vi "Main.vi"() -> ()   [LabVIEW 2015]
doc: "Use this template to build a producer/consumer design pattern with events to produce queue items. Use this design pattern instead of the User Interface Event Handler pattern for user interfaces when you want to execute code asynchronously in response to an event without slowing the user interface responsiveness."
uses:
  Typedef/JSONCluster.ctl
  Typedef/Zone Data.ctl
  <vilib>/Rock Robotics/WPI/Camera/WPI_CameraSettings Read MJPG.ctl
  <vilib>/Rock Robotics/WPI/Camera/WPI_CameraImageSize.ctl
  <vilib>/LVH/i3 JSON/i3-json.lvlib
panel:
  in  "Match List":i32(listbox)
  out "Tab":enum32{"JSON", "Field", "Match"}(tab)
  in  "Autosave CSV":bool=TRUE
  out "JSON":string
  in  "JSON Tree":string(tree)
  in  "Field Setup":bool
  in  "Save As Button":bool
  in  "Save Button":bool
  in  "Scan":bool
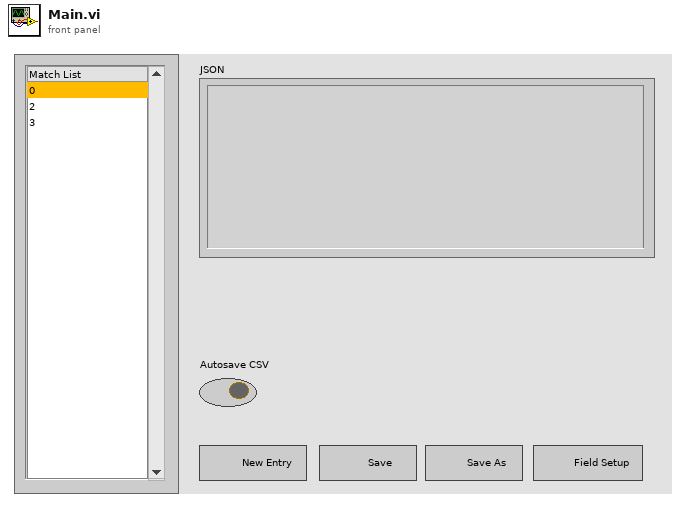
[diagram p1: front panel]
types:
  T1 = typedef "JSONCluster.ctl" = cluster{"preMatchData":cluster{"teamNumber":i32, "matchNumber":i32, "defenses":cluster{"blue1":string, "blue2":string, "blue3":string, "blue4":string, "blue5":string, "red1":string, "red2":string, "red3":string, "red4":string, "red5":string}}, "matchData":cluster{"name":string, "value":string, "items":cluster{"x":i32, "y":i32}[]}[], "matchComments":cluster{"matchComments":string, "lastComments":string}}
  T2 = typedef "Zone Data.ctl" = cluster{"Rect":cluster{"left":i16, "top":i16, "right":i16, "bottom":i16}, "Replace Values":cluster{"key":string, "value":string}[], "Name":string}
  T3 = cluster{"JSON":string, "JSONCluster":T1, "Cancelled":bool, "JSON Path":path, "CSV Path":path, "Zones":T2[]}
  T4 = typedef "WPI_CameraSettings Read MJPG.ctl" = cluster{"fps":i32, "compression":i32, "Image Size":T5}
  T5 = typedef "WPI_CameraImageSize.ctl" = enum16{"640x480", "320x240", "160x120", "Custom"}
  T6 = cluster{"teamNumber":i32, "matchNumber":i32, "defenses":cluster{"blue1":string, "blue2":string, "blue3":string, "blue4":string, "blue5":string, "red1":string, "red2":string, "red3":string, "red4":string, "red5":string}}
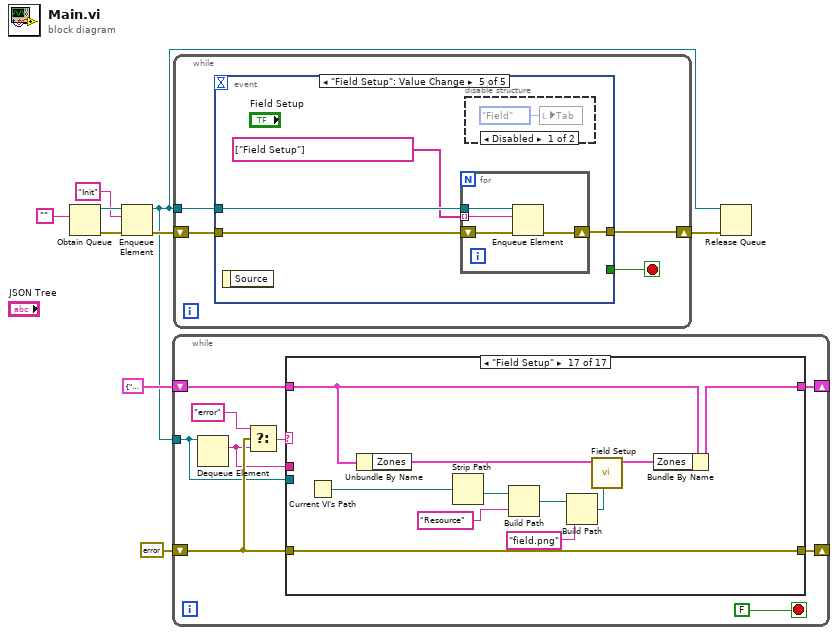
[diagram p0: block diagram]
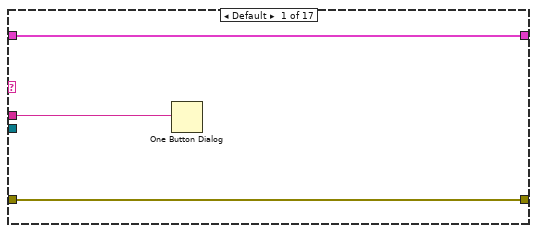
[diagram p2: hidden frame]
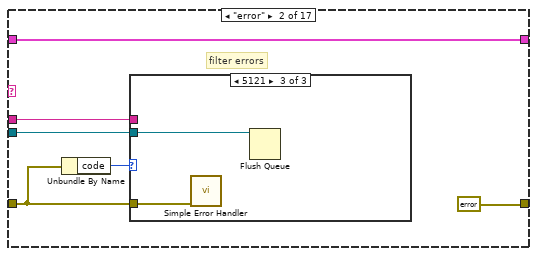
[diagram p3: hidden frame]
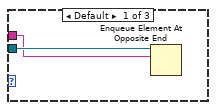
[diagram p4: hidden frame]
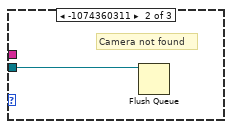
[diagram p5: hidden frame]
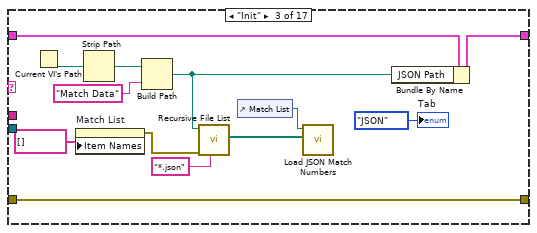
[diagram p6: hidden frame]
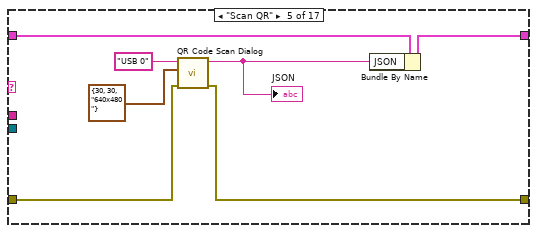
[diagram p8: hidden frame]
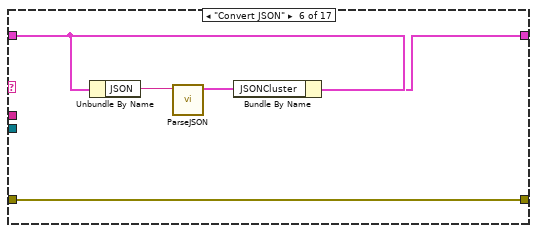
[diagram p9: hidden frame]
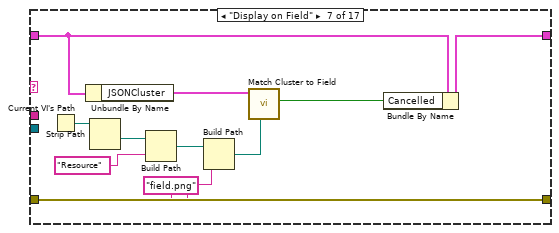
[diagram p10: hidden frame]
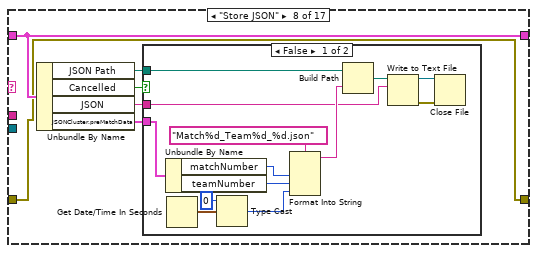
[diagram p11: hidden frame]
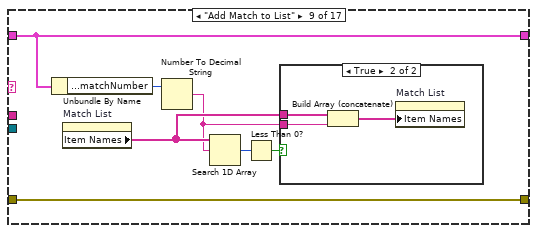
[diagram p13: hidden frame]
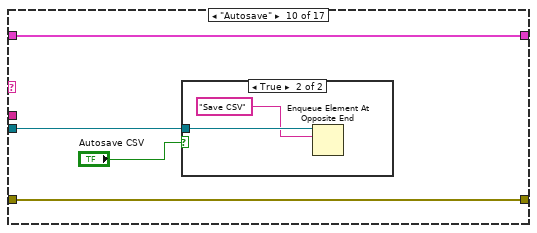
[diagram p15: hidden frame]
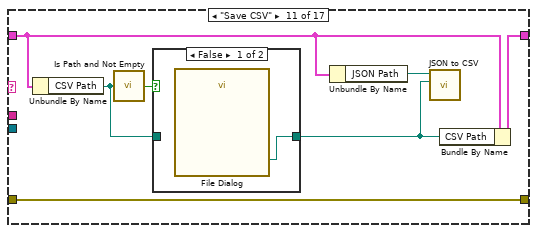
[diagram p17: hidden frame]
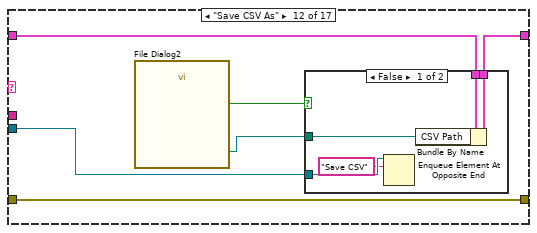
[diagram p19: hidden frame]
diagram:
  n1 = Obtain Queue(element data type="" ("data")) -> (queue out=w4:refnum<queue>, error out=w9:errorcluster)  [unwired: 4 in, 1 out]
  n2 = Enqueue Element(queue=w4, element="Init", error in (no error)=w9) -> (queue out=w3:refnum<queue>, error out=w5:errorcluster)  [unwired: 1 in, 1 out]
  n3 = while {
    tunnel: w3 -> [w10]
    shift-right: [w16] -> _
    shift-left: T3 {"JSON"="", "JSONCluster"={"preMatchData"={"teamNumber"=0, "matchNumber"=0, "defenses"={"blue1"="", "blue2"="", "blue3"="", "blue4"="", "blue5"="", "red1"="", "red2"="", "red3"="", "red4"="", "red5"=""}}, "matchData"=[], "matchComments"={"matchComments"="", "lastComments"=""}}, "Cancelled"=FALSE, "JSON Path"=path "", "CSV Path"=path "", "Zones"=[]} -> [w17]
    shift-right: [w13] -> _
    shift-left: errorcluster {"status"=FALSE, "code"=0, "source"=""} ("error out") -> [w12]
    stop <- FALSE stop-if-true
    n4 = Dequeue Element(queue=w10) -> (element=w11:string)  [unwired: 2 in, 3 out]
    n5 = Select(t="error", s=w12, f=w11) -> (s? t:f=w15:string)
    n6 = case shown="\"Field Setup\"" w15 {
      tunnel: w17 -> [w21 w27 w45 w47 w52 w58 w69 w76 w96 w103 w108 w119 w128 w138 w145 w147 w157]
      tunnel: [w21 w27 w44 w47 w51 w57 w68 w76 w96 w103 w107 w118 w128 w140 w145 w147 w155] -> w16
      tunnel: [w20 errorcluster {"status"=FALSE, "code"=0, "source"=""} ("error out") w38 w46 w49 w55 w66 w71 w90 w102 w112 w120 w127 w129 w142 w146 w158] -> w13
      tunnel: w12 -> [w20 w25 w38 w46 w48 w55 w66 w71 w90 w102 w112 w120 w127 w130 w143 w146 w158]
      tunnel: w11 -> [w19 w22 _ _ _ _ _ _ _ _ _ _ _ _ _ _ _]
      tunnel: w10 -> [_ w23 _ _ _ _ _ _ _ w101 _ w115 _ _ _ _ _]
      frame Default {
        n7 = One Button Dialog(message=w19) -> ()  [unwired: 1 in, 1 out]
      }
      frame "error" {
        # "filter errors"
        n8 = Unbundle By Name(w25) -> ("code"=w24:i32)
        n9 = case shown="5121" w24 {
          tunnel: w25 -> [_ _ w31]
          tunnel: w23 -> [w29 w30 w32]
          tunnel: w22 -> [w28 _ _]
          frame Default {
            n10 = Enqueue Element At Opposite End(queue=w29, element=w28) -> ()  [unwired: 2 in, 3 out]
          }
          frame -1074360311 {
            # "Camera not found"
            n11 = Flush Queue(queue=w30) -> ()  [unwired: 1 in, 3 out]
          }
          frame 5121 {
            n12 = call <vilib>:"Simple Error Handler.vi"("error in (no error)"=w31) -> ()  [unwired: 4 in, 5 out]
            n13 = Flush Queue(queue=w32) -> ()  [unwired: 1 in, 3 out]
          }
        }
      }
      frame "Init" {
        n14 = Current VI's Path() -> (path=w37:path)
        n15 = property on="Match List" class="LstBox (strict)"("Item Names"=string[] []) -> (error out=w35:errorcluster)  [unwired: 2 in, 1 out]
        n16 = Strip Path(path=w37) -> (stripped path=w34:path)  [unwired: 1 out]
        n17 = Build Path(base path=w34, name or relative path="Match Data") -> (appended path=w42:path)
        n18 = call <vilib>:"Recursive File List.vi"("pattern"="*.json", "error in (no error)"=w35, "Folder Path"=w42) -> ("All Files in Dir"=w41:path[])  [unwired: 4 in, 4 out]
        n19 = control-ref of="Match List"() -> (w40:refnum<vi>)
        n20 = call "Load JSON Match Numbers.vi"("All Files in Dir"=w41, "ListBox in"=w40) -> ()  [unwired: 10 in]
        n21 = Bundle By Name(cluster=w45, "JSON Path"=w42) -> (w44:T3)
        "Tab" <- enum32{"JSON", "Field", "Match"}."JSON" ("Tab")
      }
      frame "/** QR Code Handle**/" {
      }
      frame "Scan QR" {
        n22 = call "QR Code Scan Dialog.vi"("error in (no error)"=w48, "Camera Settings"=T4 {"fps"=30, "compression"=30, "Image Size"=enum."640x480"}, "Camera Address"="USB 0") -> ("error out"=w49:errorcluster, "Output"=w50:string)  [unwired: 7 in]
        "JSON" <- w50
        n23 = Bundle By Name(cluster=w52, "JSON"=w50) -> (w51:T3)
      }
      frame "Convert JSON" {
        n24 = Unbundle By Name(w58) -> ("JSON"=w59:string)
        n25 = call "ParseJSON.vi"("JSON String"=w59) -> ("JSONCluster"=w56:T1)  [unwired: 9 in, 1 out]
        n26 = Bundle By Name(cluster=w58, "JSONCluster"=w56) -> (w57:T3)
      }
      frame "Display on Field" {
        n27 = Current VI's Path() -> (path=w64:path)
        n28 = Unbundle By Name(w69) -> ("JSONCluster"=w70:T1)
        n29 = Strip Path(path=w64) -> (stripped path=w65:path)  [unwired: 1 out]
        n30 = Build Path(base path=w65, name or relative path="Resource") -> (appended path=w61:path)
        n31 = Build Path(base path=w61, name or relative path="field.png") -> (appended path=w60:path)
        n32 = call "Match Cluster to Field.vi"("path to png file"=w60, "JSONCluster"=w70) -> ("Cancelled?"=w67:bool)  [unwired: 8 in, 1 out]
        n33 = Bundle By Name(cluster=w69, "Cancelled"=w67) -> (w68:T3)
      }
      frame "Store JSON" {
        n34 = Unbundle By Name(w76) -> ("JSON Path"=w72:path, "Cancelled"=w75:bool, "JSON"=w74:string, "JSONCluster.preMatchData"=w73:T6)
        n35 = case shown="False" w75 {
          tunnel: w74 -> [w79 _]
          tunnel: w73 -> [w89 _]
          tunnel: w72 -> [w82 _]
          frame False {
            n36 = Unbundle By Name(w89) -> ("matchNumber"=w87:i32, "teamNumber"=w88:i32)
            n37 = Get Date/Time In Seconds() -> (seconds since 1Jan1904=w85:timestamp)
            n38 = Type Cast(type=i64 0, x=w85) -> (*(type *) &x=w83:i64)
            n39 = Format Into String(format string="Match%d_Team%d_%d.json", w87, w88, w83) -> (resulting string=w81:string)  [unwired: 2 in, 1 out]
            n40 = Build Path(base path=w82, name or relative path=w81) -> (appended path=w80:path)
            n41 = Write to Text File(file (use dialog)=w80, text=w79) -> (refnum out=w77:refnum<file>, error out=w78:errorcluster)  [unwired: 2 in, 1 out]
            n42 = Close File(refnum=w77, error in=w78) -> ()  [unwired: 2 out]
          }
          frame True {
          }
        }
      }
      frame "Add Match to List" {
        n43 = Unbundle By Name(w96) -> ("JSONCluster.preMatchData.matchNumber"=w95:i32)
        n44 = property on="Match List" class="LstBox (strict)"() -> ("Item Names"=w92:string[])  [unwired: 2 in, 2 out]
        n45 = Number To Decimal String(number=w95) -> (decimal integer string=w91:string)  [unwired: 1 in]
        n46 = Search 1D Array(1D array=w92, element=w91) -> (index of element=w94:i32)  [unwired: 1 in]
        n47 = Less Than 0?(x=w94) -> (x < 0?=w93:bool)
        n48 = case shown="True" w93 {
          tunnel: w92 -> [_ w99]
          tunnel: w91 -> [_ w98]
          frame False {
          }
          frame True {
            n49 = Build Array (concatenate)(w99, w98) -> (w97:string[])
            n50 = property on="Match List" class="LstBox (strict)"("Item Names"=w97) -> ()  [unwired: 2 in, 2 out]
          }
        }
      }
      frame "Autosave" {
        n51 = case shown="True" "Autosave CSV" {
          tunnel: w101 -> [_ w105]
          frame False {
          }
          frame True {
            n52 = Enqueue Element At Opposite End(queue=w105, element="Save CSV") -> ()  [unwired: 2 in, 3 out]
          }
        }
      }
      frame "Save CSV" {
        n53 = Unbundle By Name(w108) -> ("CSV Path"=w110:path)
        n54 = call <vilib>:"Is Path and Not Empty.vi"("path"=w110) -> ("Is Path and Not Empty?"=w111:bool)  [unwired: 4 in]
        n55 = case shown="False" w111 {
          tunnel: [w113 w114] -> w106
          tunnel: w110 -> [_ w114]
          frame False {
            n56 = call "File Dialog"() -> ("selected path"=w113:path)  [unwired: 12 in, 3 out]
          }
          frame True {
          }
        }
        n57 = Unbundle By Name(w108) -> ("JSON Path"=w109:path)
        n58 = call "JSON to CSV.vi"("CSV File"=w106, "JSON Path"=w109) -> ()  [unwired: 10 in]
        n59 = Bundle By Name(cluster=w108, "CSV Path"=w106) -> (w107:T3)
      }
      frame "Save CSV As" {
        n60 = call "File Dialog2"() -> ("selected path"=w117:path, "cancelled"=w116:bool)  [unwired: 12 in, 2 out]
        n61 = case shown="False" w116 {
          tunnel: w119 -> [w125 w126]
          tunnel: [w124 w126] -> w118
          tunnel: w117 -> [w123 _]
          tunnel: w115 -> [w122 _]
          frame False {
            n62 = Enqueue Element At Opposite End(queue=w122, element="Save CSV") -> ()  [unwired: 2 in, 3 out]
            n63 = Bundle By Name(cluster=w125, "CSV Path"=w123) -> (w124:T3)
          }
          frame True {
          }
        }
      }
      frame "/***Match Tab***/" {
      }
      frame "Set Active JSON" {
        n64 = Unbundle By Name(w138) -> ("JSON Path"=w137:path)
        n65 = call <vilib>:"Recursive File List.vi"("pattern"="*.json", "Folder Path"=w137) -> ("All Files in Dir"=w136:path[])  [unwired: 5 in, 4 out]
        n66 = Index Array(array=w136, index="Match List") -> (element=w134:path)
        n67 = Read from Text File(file (use dialog)=w134, error in=w130) -> (refnum out=w132:refnum<file>, text=w133:string, error out=w131:errorcluster)  [unwired: 2 in, 1 out]
        n68 = Close File(refnum=w132, error in=w131) -> (error out=w129:errorcluster)  [unwired: 1 out]
        n69 = Bundle By Name(cluster=w138, "JSON"=w133) -> (w140:T3)
      }
      frame "Display Entry on Tree" {
        n70 = Unbundle By Name(w145) -> ("JSON"=w144:string)
        n71 = control-ref of="JSON Tree"() -> (w141:refnum<vi>)
        n72 = call <vilib>:"JSON Tree View.vi"("error in (no error)"=w143, "JSON Tree Expanded Reference"=w141, "JSON Tree"=w144) -> ("error out"=w142:errorcluster)  [unwired: 7 in, 1 out]
      }
      frame "/** Field Settings **/" {
      }
      frame "Field Setup" {
        n73 = Current VI's Path() -> (path=w152:path)
        n74 = Unbundle By Name(w157) -> ("Zones"=w156:T2[])
        n75 = Strip Path(path=w152) -> (stripped path=w153:path)  [unwired: 1 out]
        n76 = Build Path(base path=w153, name or relative path="Resource") -> (appended path=w149:path)
        n77 = Build Path(base path=w149, name or relative path="field.png") -> (appended path=w148:path)
        n78 = call "Field Setup.vi"("path to png file"=w148, "Zones In"=w156) -> ("Zones Out"=w154:T2[])  [unwired: 8 in, 1 out]
        n79 = Bundle By Name(cluster=w157, "Zones"=w154) -> (w155:T3)
      }
    }
  }
  n80 = while {
    shift-right: [w159] -> w8
    shift-left: w5 -> [w161]
    tunnel: w3 -> [w162]
    stop <- w160 stop-if-true
    n81 = event shown="[4] \"Field Setup\": Value Change" {
      selector: _ -> [_ _ _ _ _]
      dyn-events: _ -> [_ _ _ _ _]
      timeout: _ -> [_ _ _ _ _]
      tunnel: w162 -> [w168 w176 w180 w182 w191]
      tunnel: w161 -> [w167 w175 w179 w183 w192]
      tunnel: [w166 w173 w177 w184 w193] -> w159
      tunnel: [FALSE _ _ _ _] -> w160
      event "Scan": Value Change {
        n82 = event-data() -> ()  [unwired: 1 in, 1 out]
        n83 = for {
          tunnel: w168 -> [w172]
          tunnel: string[] ["Scan QR", "Convert JSON", "Display on Field", "Store JSON", "Add Match to List", "Autosave"] -> [w169] mode=indexing
          shift-right: [w170] -> w166
          shift-left: w167 -> [w171]
          n84 = Enqueue Element(queue=w172, element=w169, error in (no error)=w171) -> (error out=w170:errorcluster)  [unwired: 1 in, 2 out]
        }
        n85 = local write "Tab"(enum32{"JSON", "Field", "Match"}."JSON" ("Tab")) -> ()
      }
      event "Save Button": Value Change {
        n86 = event-data() -> ()  [unwired: 1 in, 1 out]
        n87 = Enqueue Element(queue=w176, element="Save CSV", error in (no error)=w175) -> (error out=w173:errorcluster)  [unwired: 1 in, 2 out]
      }
      event "Save As Button": Value Change {
        n88 = event-data() -> ()  [unwired: 1 in, 1 out]
        n89 = Enqueue Element(queue=w180, element="Save CSV As", error in (no error)=w179) -> (error out=w177:errorcluster)  [unwired: 1 in, 2 out]
      }
      event "Match List": Value Change; "Match List": Mouse Up {
        n90 = event-data() -> ()  [unwired: 1 in, 1 out]
        n91 = for {
          tunnel: w182 -> [w189]
          tunnel: string[] ["Set Active JSON", "Display Entry on Tree"] -> [w186] mode=indexing
          shift-right: [w187] -> w184
          shift-left: w183 -> [w188]
          n92 = Enqueue Element(queue=w189, element=w186, error in (no error)=w188) -> (error out=w187:errorcluster)  [unwired: 1 in, 2 out]
        }
        n93 = local write "Tab"(enum32{"JSON", "Field", "Match"}."Match" ("Tab")) -> ()
      }
      event "Field Setup": Value Change {
        n94 = event-data() -> ()  [unwired: 1 in, 1 out]
        n95 = for {
          tunnel: w191 -> [w198]
          tunnel: string[] ["Field Setup"] -> [w195] mode=indexing
          shift-right: [w196] -> w193
          shift-left: w192 -> [w197]
          n96 = Enqueue Element(queue=w198, element=w195, error in (no error)=w197) -> (error out=w196:errorcluster)  [unwired: 1 in, 2 out]
        }
        n97 = disable-structure shown="Disabled" {
          frame Disabled {
            n98 = local write "Tab"(enum32{"JSON", "Field", "Match"}."Field" ("Tab")) -> ()
          }
          frame Enabled {
          }
        }
      }
    }
  }
  n99 = Release Queue(queue=w3, error in (no error)=w8) -> ()  [unwired: 1 in, 3 out]
